vi "LatchError_20230502.vi"(10 "error in (no error)":errorcluster, 11 "data":dbl[][](array[numeric])) -> (2 "error out":errorcluster)   [LabVIEW 2021]
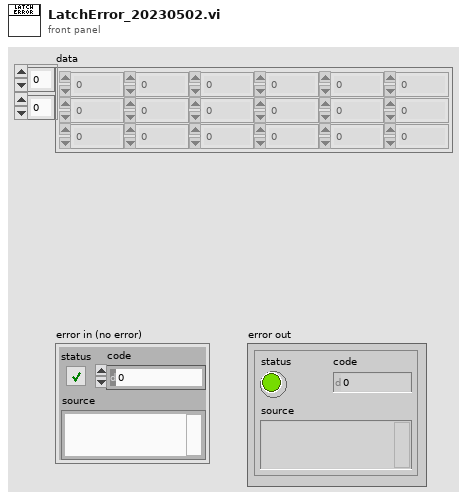
[diagram p1: front panel]
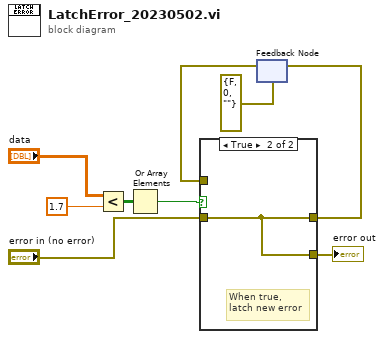
[diagram p0: block diagram]
diagram:
  n1 = Less?(x="data", y=1.7) -> (x < y?=w8:bool[][])
  n2 = Or Array Elements(Boolean array=w8) -> (logical OR=w5:bool)
  n3 = feedback #1(errorcluster {"status"=FALSE, "code"=0, "source"=""} ("error in (no error)")) -> (w2:errorcluster)
  n4 = case shown="True" w5 {
    tunnel: "error in (no error)" -> [_ w11]
    tunnel: [w10 w11] -> w4
    tunnel: [w10 w11] -> w3
    tunnel: w2 -> [w10 _]
    frame False {
      # "When false,\npreserve previous\nerror"
    }
    frame True {
      # "When true,\nlatch new error"
    }
  }
  "error out" <- w3
  n5 = feedback-in #1(w4) -> ()
